vi "CRYImport From File.vi"   [LabVIEW 2013]
uses:
  CRYMainGlobal.vi
panel:
  # "Open All Data(Curves, Values,Results, Waveforms)"
types:
  T1 = cluster{"pattern label":string, "pattern":string}
  T2 = cluster{"pattern label":string, "pattern":string}[]
  T3 = enum16{"OK", "Yes", "YesNo", "YesNoCancel", "ReplaceAppend"}
  T4 = enum16{"Left Button", "Center Button", "Right Button", "Window Close"}
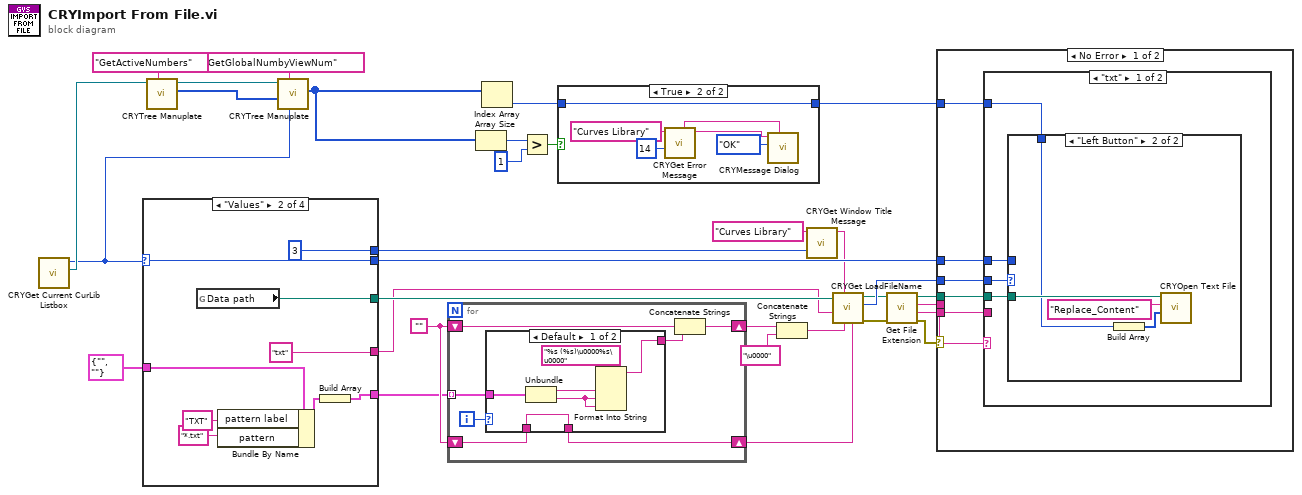
[diagram p0: block diagram]
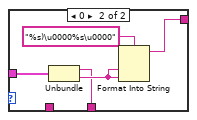
[diagram p6: hidden frame]
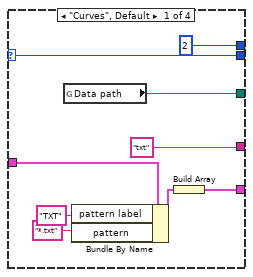
[diagram p7: hidden frame]
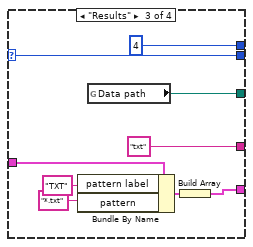
[diagram p8: hidden frame]
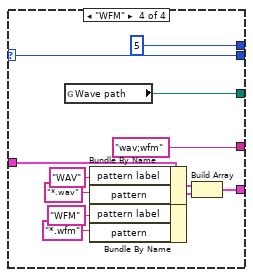
[diagram p9: hidden frame]
diagram:
  w19 = ""
  n1 = call "CRYGet Current CurLib Listbox.vi"() -> ("CurLib Tree"=w6:refnum<vi>, "Type"=w1:enum16{"Curves", "Values", "Results", "WFM"})  [unwired: 9 in, 1 out]
  n2 = case shown="\"Values\"" w1 {
    selector: w1 -> [w33 w50 w59 w71]
    tunnel: [w41 w49 w58 w70] -> w31
    tunnel: [w33 w50 w59 w71] -> w30
    tunnel: [2 ("Error No") 3 ("Error No") 4 ("Error No") 5 ("Error No")] -> w23
    tunnel: T1 {"pattern label"="", "pattern"=""} ("File Types") -> [w36 w44 w53 w62]
    tunnel: [w35 w43 w52 w61] -> w17
    tunnel: ["txt" ("pattern (all files)") "txt" ("pattern (all files)") "txt" ("pattern (all files)") "wav;wfm" ("pattern (all files)")] -> w14
    frame "Curves", Default {
      n3 = global read "CRYMainGlobal.vi" "Data path"() -> (w41:path)
      n4 = Bundle By Name(cluster=w36, "pattern label"="TXT" ("pattern (all files)"), "pattern"="*.txt" ("pattern (all files)")) -> (w39:T1)
      n5 = Build Array(w39) -> (w35:T2)
    }
    frame "Values" {
      n6 = global read "CRYMainGlobal.vi" "Data path"() -> (w49:path)
      n7 = Bundle By Name(cluster=w44, "pattern label"="TXT" ("pattern (all files)"), "pattern"="*.txt" ("pattern (all files)")) -> (w47:T1)
      n8 = Build Array(w47) -> (w43:T2)
    }
    frame "Results" {
      n9 = Bundle By Name(cluster=w53, "pattern label"="TXT" ("pattern (all files)"), "pattern"="*.txt" ("pattern (all files)")) -> (w56:T1)
      n10 = global read "CRYMainGlobal.vi" "Data path"() -> (w58:path)
      n11 = Build Array(w56) -> (w52:T2)
    }
    frame "WFM" {
      n12 = global read "CRYMainGlobal.vi" "Wave path"() -> (w70:path)
      n13 = Bundle By Name(cluster=w62, "pattern label"="WAV" ("pattern (all files)"), "pattern"="*.wav" ("pattern (all files)")) -> (w66:T1)
      n14 = Bundle By Name(cluster=w62, "pattern label"="WFM" ("pattern (all files)"), "pattern"="*.wfm" ("pattern (all files)")) -> (w65:T1)
      n15 = Build Array(w66, w65) -> (w61:T2)
    }
  }
  n16 = call "CRYTree Manuplate.vi"("sAction"="GetActiveNumbers", "Tree in"=w6) -> ("nData Out"=w3:i32[], "Tree Out"=w4:refnum<vi>)  [unwired: 6 in, 2 out]
  n17 = call "CRYTree Manuplate.vi"("Type"=w1, "sAction"="GetGlobalNumbyViewNum", "nData"=w3, "Tree in"=w4) -> ("nData Out"=w2:i32[])  [unwired: 4 in, 3 out]
  n18 = for {
    tunnel: w17 -> [w78] mode=indexing
    shift-right: [w77] -> w21
    shift-left: w19 -> [w76]
    shift-right: [w73] -> w16
    shift-left: w19 -> [w72]
    i -> [w75]
    n19 = case shown="Default" w75 {
      tunnel: w78 -> [w84 w89]
      tunnel: [w80 w86] -> w74
      tunnel: [w79 w85] -> w73
      tunnel: w72 -> [w79 _]
      frame Default {
        n20 = Unbundle(w84) -> ("pattern label"=w83:string, "pattern"=w81:string)
        n21 = Format Into String(format string="%s (%s)\u0000%s\u0000", w83, w81, w81) -> (resulting string=w80:string)  [unwired: 2 in, 1 out]
      }
      frame 0 {
        n22 = Unbundle(w89) -> ("pattern label"=w85:string, "pattern"=w87:string)
        n23 = Format Into String(format string="%s)\u0000%s\u0000", w87, w87) -> (resulting string=w86:string)  [unwired: 2 in, 1 out]
      }
    }
    n24 = Concatenate Strings(w76, w74) -> (w77:string)
  }
  n25 = Array Size(array=w2) -> (size(s)=w13:i32)
  n26 = Index Array(array=w2) -> (element=w10:i32)  [unwired: 1 in]
  n27 = Greater?(x=w13, y=1) -> (0:w11:bool)
  n28 = case shown="True" w11 {
    tunnel: [w90 w91] -> w9
    tunnel: w10 -> [w90 w91]
    frame False {
    }
    frame True {
      n29 = call "CRYGet Error Message.vi"("Error No"=14, "Kind"="Curves Library") -> ("Message"=w93:string, "Window Title"=w92:string)  [unwired: 4 in, 4 out]
      n30 = call "CRYMessage Dialog.vi"("Window Title"=w92, "YesNoCancel"=T3."OK", "Message Content"=w93) -> ()  [unwired: 7 in, 2 out]
    }
  }
  n31 = Concatenate Strings(w21, "\u0000" ("format string")) -> (w15:string)
  n32 = call "CRYGet Window Title Message.vi"("No"=w23, "Kind"="Curves Library") -> ("Multibyte String"=w22:string)  [unwired: 4 in, 5 out]
  n33 = call "CRYGet LoadFileName.vi"("pattern label"=w16, "pattern (all files)"=w15, "TitleName"=w22, "Category Name"=w14, "Start path"=w31) -> ("error out"=w27:errorcluster, "Which Button?"=w32:T4, "Path"=w29:path)  [unwired: 3 in, 1 out]
  n34 = call <vilib>:"Get File Extension.vi"("error in (no error)"=w27, "file"=w29) -> ("error out"=w8:errorcluster, "filename without extension"=w26:string, "lowercase file extension"=w25:string, "dup file"=w28:path)  [unwired: 6 out]
  n35 = case shown="No Error" w8 {
    tunnel: w32 -> [w102 _]
    tunnel: w30 -> [w101 _]
    tunnel: w28 -> [w100 _]
    tunnel: w26 -> [w99 _]
    tunnel: w25 -> [w98 _]
    tunnel: w9 -> [w97 _]
    frame No Error {
      n36 = case shown="\"txt\"" w98 {
        tunnel: w102 -> [w106 _]
        tunnel: w101 -> [w105 _]
        tunnel: w100 -> [w103 _]
        tunnel: w99 -> [_ _]
        tunnel: w97 -> [w104 _]
        frame "txt" {
          n37 = case shown="\"Left Button\"" w106 {
            tunnel: w103 -> [_ w109]
            tunnel: w105 -> [_ _]
            tunnel: w104 -> [_ w108]
            frame "Center Button", Default {
            }
            frame "Left Button" {
              n38 = Build Array(w108) -> (w107:i32[])
              n39 = call "CRYOpen Text File.vi"("Index"=w107, "sOption"="Replace_Content", "File Path"=w109) -> ()  [unwired: 7 in, 2 out]
            }
          }
        }
        frame Default {
        }
      }
    }
    frame Error {
    }
  }
